vi "cam0-制作槽边选框ROI.vi"(8 "产品位指向角度":sgl, 9 "槽点位":cluster{"X":sgl, "Y":sgl}, 10 "Cut基点":cluster{"X":sgl, "Y":sgl}) -> (2 "ROI Descriptor":T1 {"Contours"."Type" items=["No Selection", "Point", "Line", "Rectangle", "Oval", "Polygon", "Freehand Region", "Annulus", "Unused2", "Unused3", "Broken Line", "Freehand Line", "Rotated Rectangle"]})   [LabVIEW 2015]
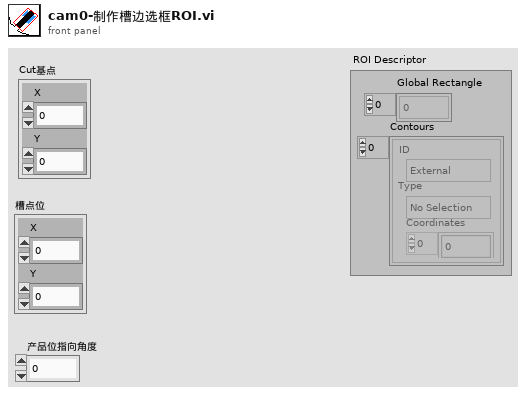
[diagram p1: front panel]
types:
  T1 = typedef "ROI Descriptor" = cluster{"Global Rectangle":i32[], "Contours":cluster{"ID":enum32{"External", "Internal"}, "Type":u32, "Coordinates":i32[]}[]}
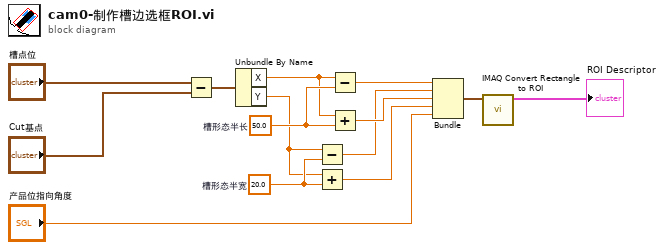
[diagram p0: block diagram]
diagram:
  w14 = sgl 50.0  # 槽形态半长
  w7 = sgl 20.0  # 槽形态半宽
  n1 = Subtract(x="槽点位", y="Cut基点") -> (x-y=w13:cluster{"X":sgl, "Y":sgl})
  n2 = Unbundle By Name(w13) -> ("X"=w5:sgl, "Y"=w6:sgl)
  n3 = Subtract(x=w6, y=w7) -> (x-y=w9:sgl)
  n4 = Add(x=w6, y=w7) -> (x+y=w11:sgl)
  n5 = Subtract(x=w5, y=w14) -> (x-y=w8:sgl)
  n6 = Add(x=w5, y=w14) -> (x+y=w10:sgl)
  n7 = Bundle(w8, w9, w10, w11, "产品位指向角度"="产品位指向角度") -> (w12:cluster{sgl, sgl, sgl, sgl, "产品位指向角度":sgl})  [unwired: 1 in]
  n8 = call "IMAQ Convert Rectangle to ROI"("Rectangle"=w12) -> ("ROI Descriptor"=→"ROI Descriptor":T1)  [unwired: 8 in, 1 out]
